vi "Configure H3611i.vi"(8 "error in (no error)":errorcluster, 10 "uWave Range Refnum":refnum<vi>, 11 "H3611i Actor in":refnum<class "H3611i Actor.lvclass">) -> (0 "error out":errorcluster, 3 "H3611i Actor out":refnum<class "H3611i Actor.lvclass">)   [LabVIEW 2018, in "H3611i.lvlib" / "H3611i Actor.lvclass"]
uses:
  H3611i Actor.lvclass
  C:/Users/dev/Documents/CODE/LabVIEW/microwaveverify/trunk/MWWL Verification/Sensor Actor/Sensor/Sensor.lvclass
  C:/Program Files (x86)/National Instruments/LabVIEW 2018/vi.lib/ActorFramework/Actor/Actor.lvclass
  H3611i Actor.lvclass/H3611i Actor.ctl
  <vilib>/ActorFramework/Actor/Actor.lvclass/Actor.ctl
  MWWL Verification/MWWL Verification Messages/Log Event Msg/Log Event Msg.lvclass/Log Event Msg.ctl
  <vilib>/ActorFramework/Message Enqueuer/Message Enqueuer.lvclass/Message Enqueuer.ctl
  <vilib>/ActorFramework/Message Enqueuer/Enqueue.vi
  MWWL Verification/MWWL Verification Messages/Log Event Msg/Log Event Msg.lvclass
  C:/Program Files (x86)/National Instruments/LabVIEW 2018/vi.lib/ActorFramework/Message/Message.lvclass
  <vilib>/Instr/_visa.llb/VISA Configure Serial Port (Instr).vi
  <vilib>/ActorFramework/Message Priority Queue/Priority Enqueue.vi
  Sensor Actor/Sensor/Sensor.lvclass
  <vilib>/ActorFramework/Actor/Actor.lvclass
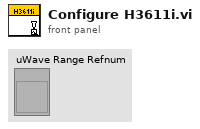
[diagram p1: front panel]
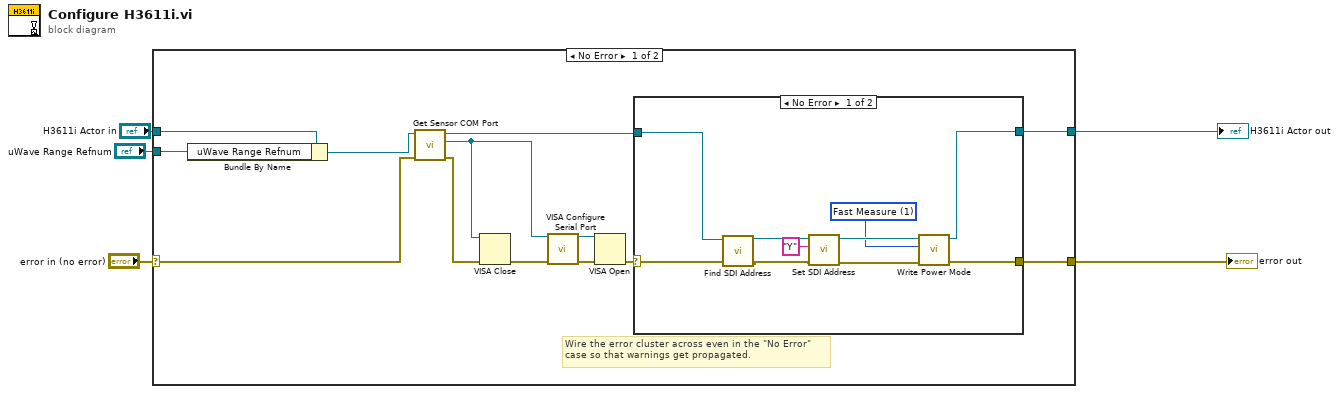
[diagram p0: block diagram]
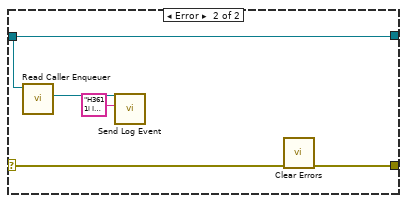
[diagram p2: hidden frame]
diagram:
  n1 = case shown="No Error" "error in (no error)" {
    selector: "error in (no error)" -> [w10 w35]
    tunnel: [w18 w35] -> w4
    tunnel: [w16 w34] -> w2
    tunnel: "H3611i Actor in" -> [w8 w34]
    tunnel: "uWave Range Refnum" -> [w7 _]
    frame No Error {
      # "Wire the error cluster across even in the \"No Error\"\ncase so that warnings get propagated."
      n2 = Bundle By Name(cluster=w8, "uWave Range Refnum"=w7) -> (w6:refnum<class "H3611i Actor.lvclass">)
      n3 = call "Get Sensor COM Port.vi"("error in (no error)"=w10, "Sensor in"=w6) -> ("error out"=w9:errorcluster, "COM Port"=w12:refnum<visa-resource-name>, "Sensor out"=w17:refnum<class "H3611i Actor.lvclass">)  [unwired: 7 in]
      n4 = VISA Close(VISA resource name=w12, error in (no error)=w9) -> (error out=w11:errorcluster)
      n5 = call-poly "VISA Configure Serial Port"("VISA resource name"=w12, "error in (no error)"=w11) -> ("VISA resource name out"=w14:refnum<visa-resource-name>, "error out"=w13:errorcluster)  [unwired: 12 in]
      n6 = VISA Open(error in (no error)=w13, VISA resource name=w14) -> (error out=w15:errorcluster)  [unwired: 3 in, 1 out]
      n7 = case shown="No Error" w15 {
        selector: w15 -> [w25 w33]
        tunnel: [w23 w32] -> w18
        tunnel: w17 -> [w19 w29]
        tunnel: [w21 w29] -> w16
        frame No Error {
          w20 = u16 1 items=["Sleep", "Fast Measure"]
          n8 = call "Find SDI Address.vi"("error in (no error)"=w25, "H3611i Actor in"=w19) -> ("error out"=w28:errorcluster, "H3611i Actor out"=w27:refnum<class "H3611i Actor.lvclass">)  [unwired: 8 in]
          n9 = call "Set SDI Address.vi"("error in (no error)"=w28, "SDI Address"="Y", "H3611i Actor in"=w27) -> ("error out"=w24:errorcluster, "H3611i Actor out"=w22:refnum<class "H3611i Actor.lvclass">)  [unwired: 7 in]
          n10 = call "Write Power Mode.vi"("error in (no error)"=w24, "Power Mode"=w20, "H3611i Actor in"=w22) -> ("error out"=w23:errorcluster, "H3611i Actor out"=w21:refnum<class "H3611i Actor.lvclass">)  [unwired: 7 in]
        }
        frame Error {
          n11 = call <vilib>:"Read Caller Enqueuer.vi"("Actor"=w29) -> ("Caller Enqueuer"=w30:refnum<class "Message Enqueuer.lvclass">)  [unwired: 10 in]
          n12 = call "Send Log Event.vi"("Event Text"="H3611i Init  Failed.\nCLose and Re-Initialize." ("message"), "Message Enqueuer"=w30) -> ()  [unwired: 8 in, 2 out]
          n13 = call <vilib>:"Clear Errors.vi"("error in (no error)"=w33) -> ("error out"=w32:errorcluster)  [unwired: 5 in, 1 out]
        }
      }
    }
    frame Error {
    }
  }
  "error out" <- w4
  "H3611i Actor out" <- w2
